vi "Main_Robot.vi"(0 "VISA resource name":refnum<visa-resource-name>="COM1", 1 "baud rate":u32=9600, 4 "data bits":u16=8 min=5 max=8 step=1, 5 "parity":u16(ring) items=["None", "Odd", "Even", "Mark", "Space"], 7 "stop bits":u16(ring)=10 items=["1.0"=10, "1.5"=15, "2.0"=20], 9 "XON Character":u8=17 format="%.0x", 14 "XOFF Character":u8=19 format="%.0x", 15 "timeout (ms)":u32=10000, 21 "End read on termination character?":bool=TRUE, 24 "termination char\n(0xA = '\\n' = LF)":u8=10 format="%.0x", 25 "Input\nbuffer size":u32=4096) -> ()   [LabVIEW 2009]
doc: "The Advanced Serial Read and Write example performs a Serial Port Read, a Serial Port Write, or a combination of these actions while setting some advanced serial features like buffer size, termination characters, and XON/XOFF flow control. The user selects the actions (read or write) on the front panel. If both are selected, the VI will write the data first, read the data and then close the VISA session that is opened to the port. \n\nThe parameters set for the serial port must match the parameters of the connected instrument or device. In this example, the bytes to read parameter specifies the number of bytes that the serial port reads. If there were more bytes at the port than the number specified in bytes to read, those bytes would not be read. Also, if you specify to read more bytes than the number of bytes actually read, you might receive a timeout error message.\n\nINSTRUCTIONS:\n1) Select the serial resource and configuration parameters (baud rate, data bits, parity, stop bits, flow control).\n2) Termination character can be enabled and set. Also, set the required input buffer size prior to running the example.\n3) Select the operations to be performed. \n4) Connect the serial port to your device. If no device is available, perform a loopback test by doing one of the following. Short pins 2 and 3 on a RS-232 cable or short pin 4 to pin 8 and pin 5 to pin 9 on a RS-485/422 cable. \n5) Run the VI to see the data read. (The \"read string\" will match the \"string to write\" if a loopback test was performed.)\n\nThis example exposes several advanced features that you may need for your application. Not all applications need all the features shown in this example. The input buffer size is likely an important setting that you want to control in your application. This example expands upon the flow control option for XON and XOFF, allowing the user to choose those control characters. The timeout parameter has been brought to the front panel so a user can specify the time period the VISA Read will wait for the number of bytes to read before timing out. Also, the user has several controls for the termination character, which is discussed later.\n\nNote that you can press the write and read buttons and change the bytes to read parameters on the fly, while the example is running. However, you must stop the example to change the other configuration parameters after the example has started running, and then run again.\n\nSet the I/O buffer size slightly higher the amount of data you expect to receive. This is very important for applications that don't use flow control, as you may lose characters if the receive buffer overflows.\n\nSetting the timeout period ensures that the operation returns with a timeout error if the operation cannot be performed in the specified time period. \n\nSome devices require a termination character in order to identify the end of command strings. Some devices send a termination character to signify the end of data to be read. \n\nThis example shows how you can end the Read operation once a termination character is detected in the buffer and/or append a termination character at the end of the Write data. To enable the Read to end on a termination character, use the VISA Configure Serial Port or use the VISA Properties Serial End Mode for Reads, Termination Character Enable, and Termination Character. To end the Write with a termination character, use the VISA Properties Serial End Mode for Writes, the Send End Enable, and Termination Character. In this example, the same termination character is used for both the Read and the Write. You can specify two different characters for your application, if desired.\n\nYour application may require specific characters for the XON/XOFF Flow Control. You can specify these characters with the VISA Properties Flow Control XOFF Character and Flow Control XON Character. Note that if the standard XON and XOFF characters are used, then decimal 17 and 19 are unavailable for data values. Remember that using flow control and setting an adequate buffer size allow you to prevent buffer overflows."
uses:
  <vilib>/Instr/_visa.llb/VISA Configure Serial Port (Instr).vi
  <vilib>/measure/madcrms.llb/Basic Averaged DC-RMS for 1 Chan.vi
  <vilib>/express/express analysis/Spectral/XNode/ExpressSpectralMeasurementsBlockNode.xnode
  <vilib>/express/express analysis/Spectral/Block/exnSpectralBlock spectral measurements peak poly.vi
  <vilib>/express/express analysis/Spectral/Block/exnSpectralBlock spectral measurements peak DDT.vi
  <vilib>/measure/NI_MAPro.lvlib
panel:
  in  "Transmit \nInterval (s)":dbl=1.0
  out "Data \nTransmit":string
  in  "I DC":dbl=1.0
  in  "Q DC":dbl=1.0
  out "Human \nDetected?":bool
  in  "Threshold":dbl=200.0
  out "Intensity":waveform(dbl)(graph)
  out "I/Q Spectrum":dynamicdata(graph)
  out "Q channel":waveform(dbl)(graph)={"t0"=timestamp(3198752920.9360003 s since 1904-01-01), "dt"=0.08500000089406967, "Y"=[0.0, 0.0, 0.0, 0.0, 0.0, 0.0, 0.0, 0.0, 0.0, 0.0, 0.0, 0.0, 0.0, 0.0, 0.0, 0.0, 0.0, 0.0, 0.0, 0.0, 0.0, 0.0, 0.0, 0.0, 0.0, 0.0, 0.0, 0.0, 0.0, 0.0, 0.0, 0.0, 0.0, 0.0, 0.0, 0.0, 0.0, 0.0, 0.0, 0.0, 0.0, 0.0, 0.0, 0.0, 0.0, 0.0, 0.0, 0.0, 0.0, 0.0, 0.0, 0.0, 0.0, 0.0, 0.0, 0.0, 0.0, 0.0, 0.0, 0.0, 0.0, 0.0913849025964737, 0.286313533782959, 0.027054062113165855, 0.019259560853242874, 0.2238655835390091, -0.08488079905509949, -0.24375496804714203, -0.09403041750192642, -0.1046101301908493, -0.17000871896743774, 0.13043256103992462, -0.18301288783550262, -0.2802070379257202, -0.05985879898071289, 0.032467812299728394, -0.06909587979316711, 0.12423869222402573, -0.13009318709373474, -0.09696193039417267, 0.13724742829799652, -0.2714601755142212, -0.3184712529182434, 0.13420049846172333, 0.05935952439904213, -0.05841037631034851, 0.2082899808883667, -0.03580809012055397, -0.22062736749649048, 0.06683129817247391, -0.15559138357639313, -0.2515611946582794, 0.05501296743750572, 0.19322194159030914, 0.14264245331287384, 0.36089611053466797, -0.06836720556020737, -0.0454566664993763, -0.0610920712351799, -0.2674013674259186, -0.22359579801559448, -0.09999596327543259, 0.049278225749731064, -0.0071744536980986595, -0.060943424701690674, 0.19243650138378143, 0.10976719856262207, 0.10197310894727707, 0.07962939888238907, 0.2600933611392975, 0.7772611379623413, 0.5951973795890808, 0.4565841257572174, 0.5391018390655518, 0.2501334249973297, -0.05727807804942131, -0.42460599541664124, -0.49300429224967957, -0.6962898373603821, -0.6063411831855774, -0.371660977602005, -0.45583224296569824, -0.3658473789691925, 0.27788665890693665, 0.13202670216560364, -0.05904369801282883, 0.19415463507175446, -0.07230788469314575]}
  out "I channel":waveform(dbl)(graph)={"t0"=timestamp(3198752920.9360003 s since 1904-01-01), "dt"=0.08500000089406967, "Y"=[0.0, 0.0, 0.0, 0.0, 0.0, 0.0, 0.0, 0.0, 0.0, 0.0, 0.0, 0.0, 0.0, 0.0, 0.0, 0.0, 0.0, 0.0, 0.0, 0.0, 0.0, 0.0, 0.0, 0.0, 0.0, 0.0, 0.0, 0.0, 0.0, 0.0, 0.0, 0.0, 0.0, 0.0, 0.0, 0.0, 0.0, 0.0, 0.0, 0.0, 0.0, 0.0, 0.0, 0.0, 0.0, 0.0, 0.0, 0.0, 0.0, 0.0, 0.0, 0.0, 0.0, 0.0, 0.0, 0.0, 0.0, 0.0, 0.0, 0.0, 0.0, 0.0913849025964737, 0.286313533782959, 0.027054062113165855, 0.019259560853242874, 0.2238655835390091, -0.08488079905509949, -0.24375496804714203, -0.09403041750192642, -0.1046101301908493, -0.17000871896743774, 0.13043256103992462, -0.18301288783550262, -0.2802070379257202, -0.05985879898071289, 0.032467812299728394, -0.06909587979316711, 0.12423869222402573, -0.13009318709373474, -0.09696193039417267, 0.13724742829799652, -0.2714601755142212, -0.3184712529182434, 0.13420049846172333, 0.05935952439904213, -0.05841037631034851, 0.2082899808883667, -0.03580809012055397, -0.22062736749649048, 0.06683129817247391, -0.15559138357639313, -0.2515611946582794, 0.05501296743750572, 0.19322194159030914, 0.14264245331287384, 0.36089611053466797, -0.06836720556020737, -0.0454566664993763, -0.0610920712351799, -0.2674013674259186, -0.22359579801559448, -0.09999596327543259, 0.049278225749731064, -0.0071744536980986595, -0.060943424701690674, 0.19243650138378143, 0.10976719856262207, 0.10197310894727707, 0.07962939888238907, 0.2600933611392975, 0.7772611379623413, 0.5951973795890808, 0.4565841257572174, 0.5391018390655518, 0.2501334249973297, -0.05727807804942131, -0.42460599541664124, -0.49300429224967957, -0.6962898373603821, -0.6063411831855774, -0.371660977602005, -0.45583224296569824, -0.3658473789691925, 0.27788665890693665, 0.13202670216560364, -0.05904369801282883, 0.19415463507175446, -0.07230788469314575]}
  out "Hiher2":u8
  out "Lower6":u8
  in  "t0":timestamp=timestamp(3198752888.296 s since 1904-01-01)
  in  "FFT":i32=256
  in  "stop":bool
  in  "flow control":u16(ring) items=["None"=0, "XON/XOFF"=1, "RTS/CTS"=2, "DTR/DSR"=4]
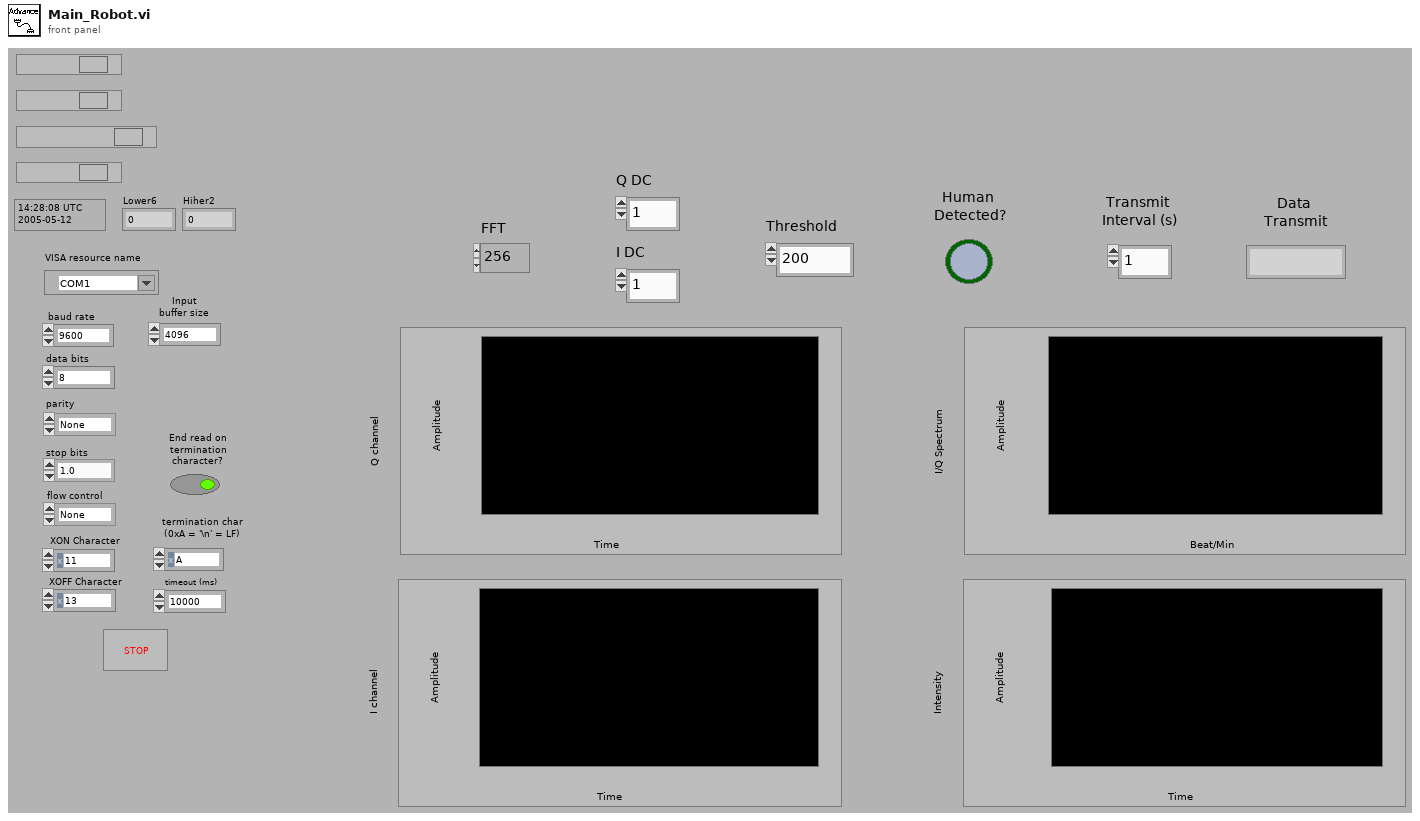
[diagram p1: front panel]
types:
  T1 = cluster{"averaging mode":u16, "weighting mode":u16, "number of averages":u32}
  T2 = cluster{"dB On (F)":bool, "unwrap phase (F)":bool, "convert to degree (F)":bool}
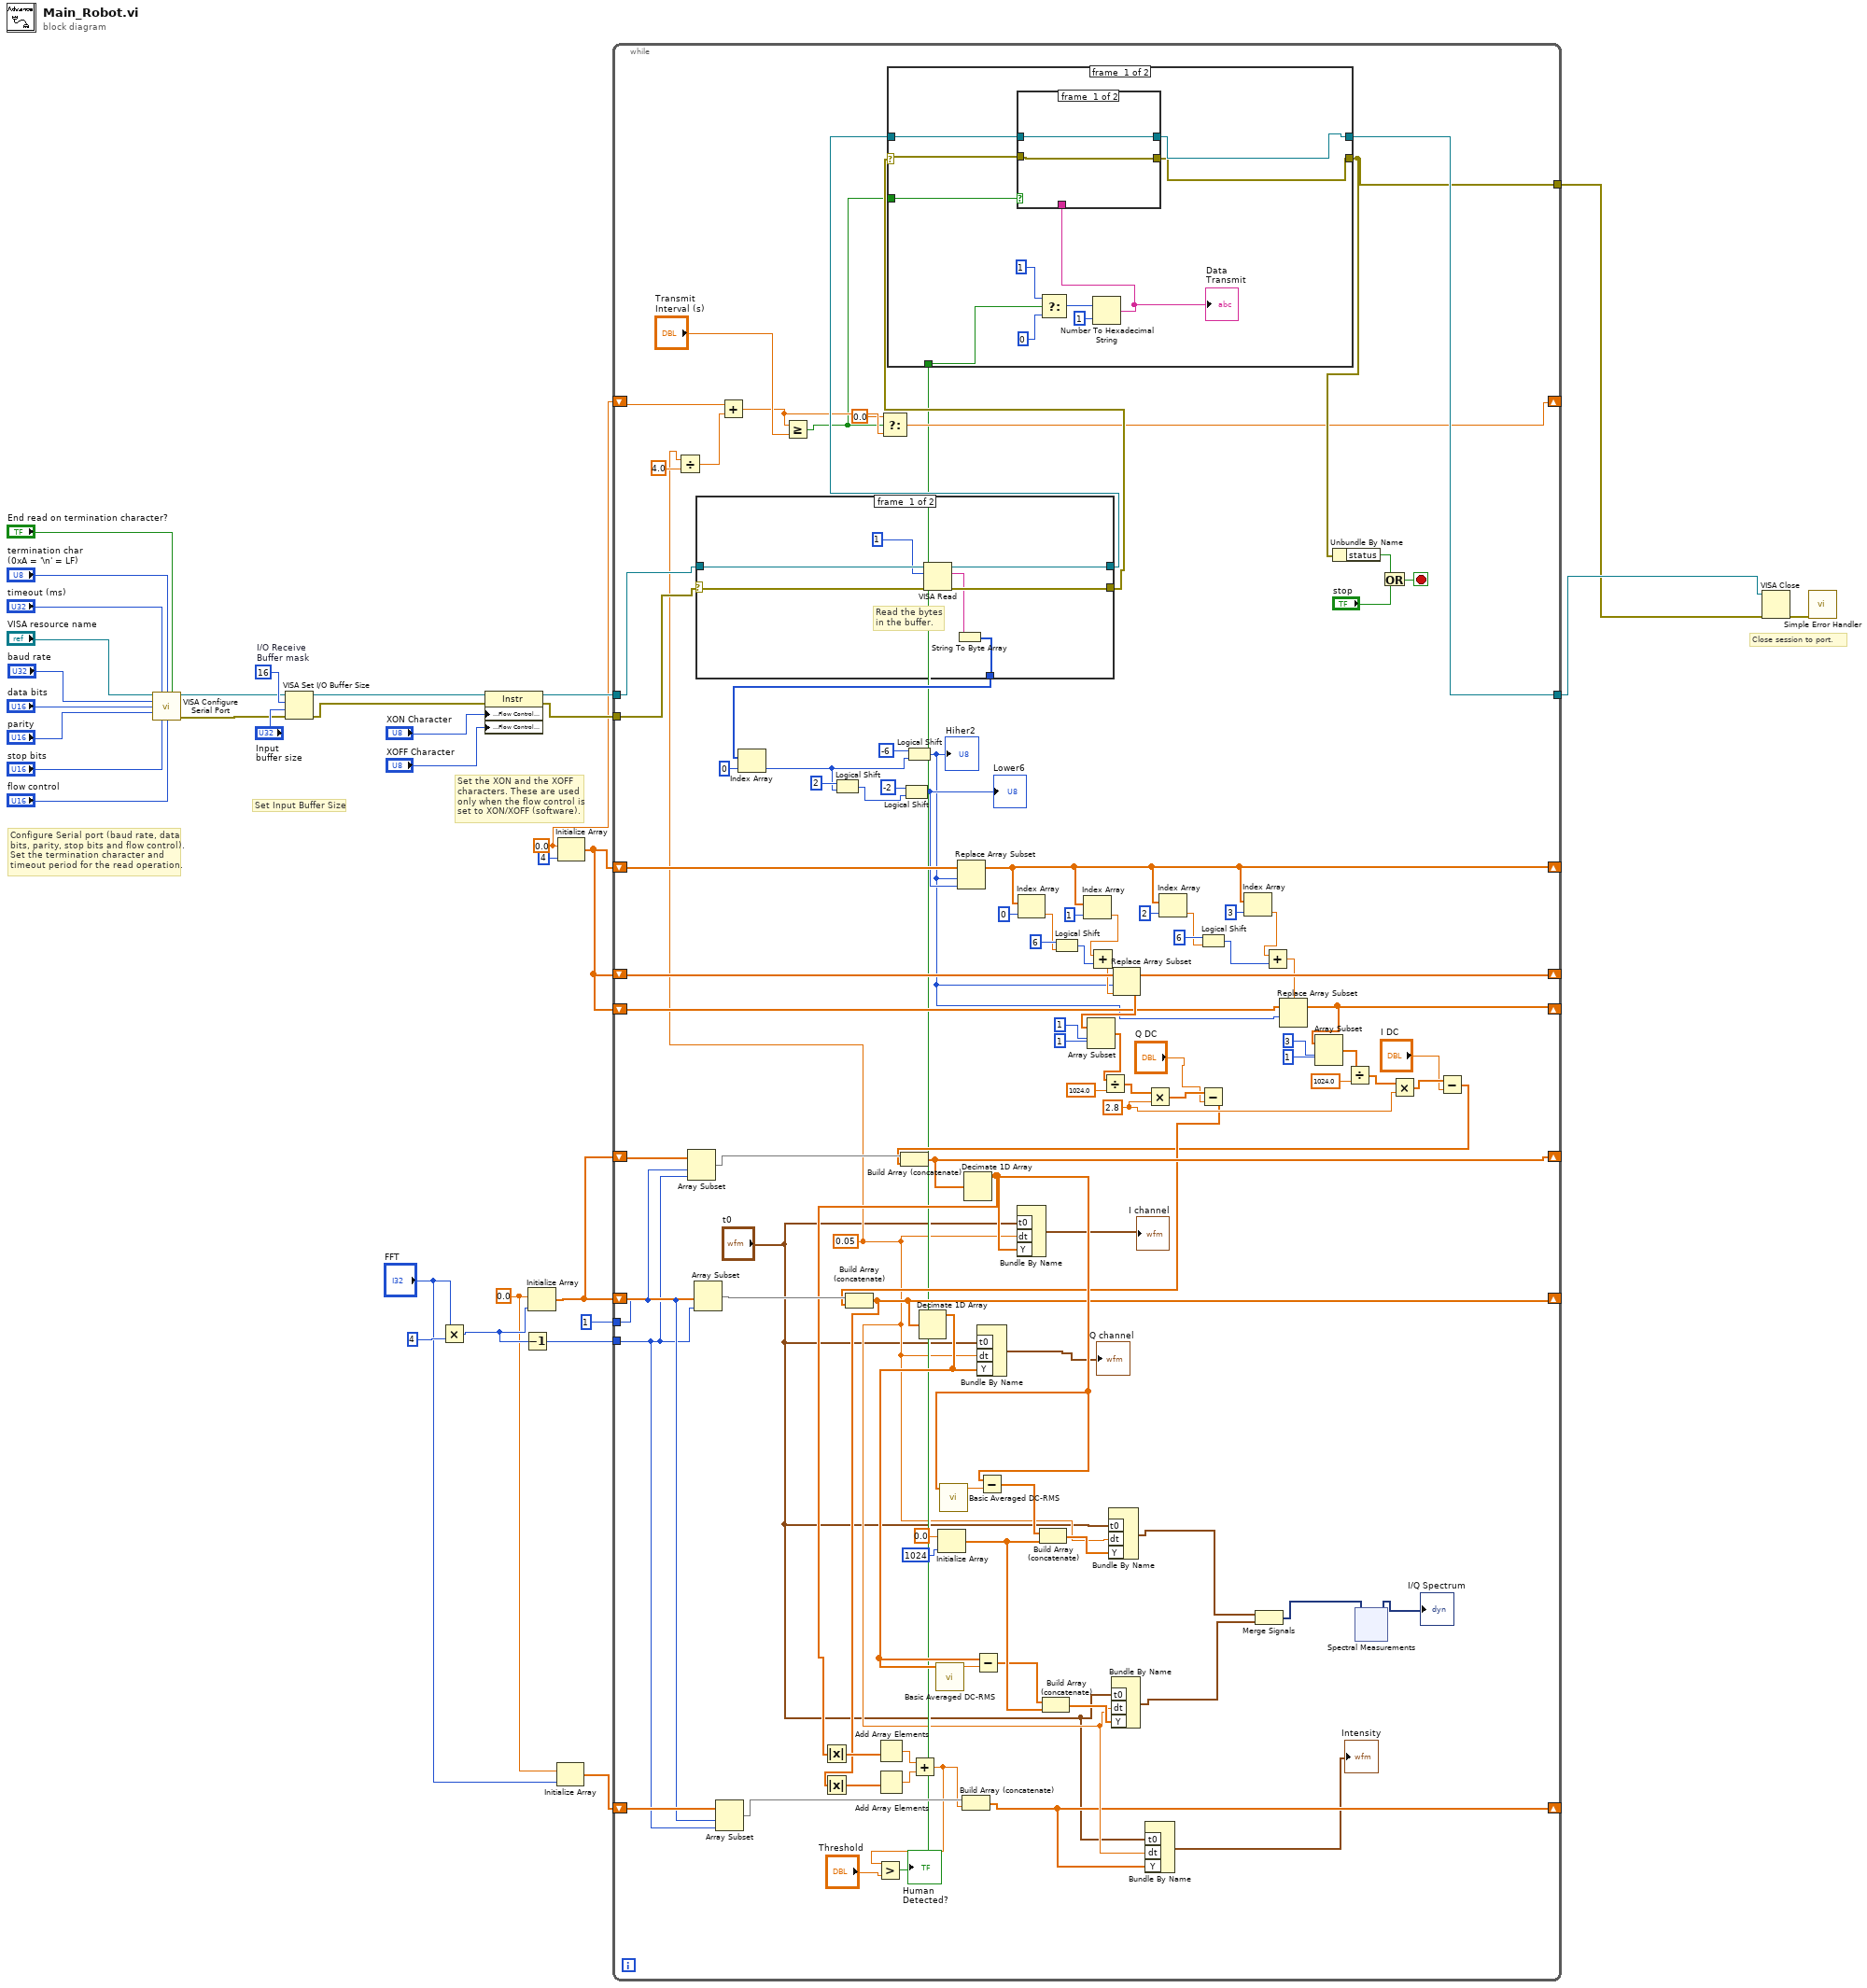
[diagram p0: block diagram]
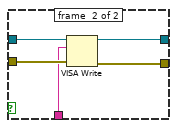
[diagram p2: hidden frame]
diagram:
  w1 = 0.0 ("element")
  w5 = 0.0 ("element")
  w26 = u16 16  # I/O Receive Buffer mask
  # "Set the XON and the XOFF\ncharacters. These are used\nonly when the flow control is\nset to XON/XOFF (software)."
  # "Configure Serial port (baud rate, data\nbits, parity, stop bits and flow control).\nSet the termination character and\ntimeout period for the read operation."
  # "Set Input Buffer Size"
  # "Close session to port."
  n1 = call-poly "VISA Configure Serial Port"("VISA resource name"="VISA resource name", "timeout (10sec)"="timeout (ms)", "termination char\n(0xA = '\\n' = LF)"="termination char\n(0xA = '\\n' = LF)", "Enable Termination\nChar (T)"="End read on termination character?", "baud rate (9600)"="baud rate", "data bits (8)"="data bits", "parity (0:none)"="parity", "stop bits (10: 1 bit)"="stop bits", "flow control (0:none)"="flow control") -> ("VISA resource name out"=w15:refnum<visa-resource-name>, "error out"=w14:errorcluster)  [unwired: 5 in]
  n2 = VISA Set I/O Buffer Size(VISA resource name=w15, mask (16)=w26, size (4096)="Input\nbuffer size", error in (no error)=w14) -> (VISA resource name out=w22:refnum<visa-resource-name>, error out=w21:errorcluster)
  n3 = Multiply(x="FFT", y=4) -> (x*y=w8:i32)
  n4 = property class="Instr"(reference=w22, error in=w21, "Serial Settings:Flow Control XON Character"="XON Character", "Serial Settings:Flow Control XOFF Character"="XOFF Character") -> (reference out=w16:refnum<visa-resource-name>, error out=w18:errorcluster)
  n5 = Decrement(x=w8) -> (x-1=w13:i32)
  n6 = Initialize Array(w5, w8) -> (w10:dbl[])
  n7 = Initialize Array(w5, "FFT") -> (w4:dbl[])
  n8 = Initialize Array(w1, 4 ("dimension size")) -> (w9:dbl[])
  n9 = while {
    tunnel: w18 -> [w53]
    tunnel: w16 -> [w54]
    tunnel: [w50] -> w3
    tunnel: w13 -> [w35]
    tunnel: 1 ("index") -> [w36]
    shift-right: [w66] -> _
    shift-left: w10 -> [w129]
    shift-right: [w117] -> _
    shift-left: w9 -> [w123]
    shift-right: [w70] -> _
    shift-left: w10 -> [w107]
    shift-right: [w99] -> _
    shift-left: w9 -> [w101]
    shift-right: [w91] -> _
    shift-left: w9 -> [w94]
    shift-right: [w39] -> _
    shift-left: w4 -> [w73]
    tunnel: [w49] -> w2
    shift-right: [w44] -> _
    shift-left: w1 -> [w48]
    stop <- w133 stop-if-true
    w78 = 2.8 ("y")
    w40 = 0.05 ("dt")
    n10 = Divide(x=w40, y=4.0) -> (x/y=w42:dbl)
    n11 = Array Subset(array=w107, index=w36, length=w35) -> (w108:dbl[])
    n12 = Array Subset(array=w129, index=w36, length=w35) -> (w131:dbl[])
    n13 = case "Read bytes from port." shown="No Error" w53 {
      selector: w53 -> [w169 w174]
      tunnel: [w171 w174] -> w51
      tunnel: [w172 w175] -> w52
      tunnel: w54 -> [w170 w175]
      tunnel: [w167 u8[] [] ("unsigned byte array")] -> w106
      frame #0 {
        # "Read the bytes\nin the buffer."
        n14 = VISA Read(VISA resource name=w170, byte count=u32 1, error in (no error)=w169) -> (VISA resource name out=w172:refnum<visa-resource-name>, read buffer=w168:string, error out=w171:errorcluster)  [unwired: 1 out]
        n15 = String To Byte Array(string=w168) -> (unsigned byte array=w167:u8[])
      }
      frame #1 {
        # "Error occurred \nreading Bytes at \nSerial Port"
      }
    }
    n16 = Array Subset(array=w73, index=w36, length=w35) -> (w72:dbl[])
    n17 = Add(x=w48, y=w42) -> (x+y=w46:dbl)
    n18 = Index Array(array=w106, index=0) -> (element=w126:u8)
    n19 = Greater Or Equal?(x=w46, y="Transmit \nInterval (s)") -> (x >= y?=w34:bool)
    n20 = Logical Shift(y=i8 2, x=w126) -> (x << y=w125:u8)
    n21 = Select(t=0.0, s=w34, f=w46) -> (s? t:f=w44:dbl)
    n22 = Logical Shift(y=i8 -2, x=w125) -> (x << y=w122:u8)
    "Lower6" <- w122
    n23 = Logical Shift(y=i8 -6, x=w126) -> (x << y=w89:u8)
    "Hiher2" <- w89
    n24 = Initialize Array(0.0 ("element"), 1024 ("dimension size")) -> (w82:dbl[])
    n25 = Replace Array Subset(array=w123, new element=w122, index=w89) -> (w117:dbl[])
    n26 = Index Array(array=w117, index=0) -> (element=w115:dbl)
    n27 = Logical Shift(y=i16 6, x=w115) -> (x << y=w111:u32)
    n28 = Index Array(array=w117, index=1) -> (element=w112:dbl)
    n29 = Add(x=w112, y=w111) -> (x+y=w100:dbl)
    n30 = Replace Array Subset(array=w101, new element=w100, index=w89) -> (w99:dbl[])
    n31 = Array Subset(array=w99, index=1, length=1) -> (w96:dbl[])
    n32 = Divide(x=w96, y=1024.0) -> (x/y=w104:dbl[])
    n33 = Multiply(x=w104, y=w78) -> (x*y=w60:dbl[])
    n34 = Index Array(array=w117, index=2) -> (element=w113:dbl)
    n35 = Logical Shift(y=i16 6, x=w113) -> (x << y=w109:u32)
    n36 = Subtract(x=w60, y="Q DC") -> (x-y=w59:dbl[])
    n37 = Build Array (concatenate)(w131, w59) -> (w66:dbl[])
    n38 = Absolute Value(x=w66) -> (abs(x)=w76:dbl[])
    n39 = Add Array Elements(numeric array=w76) -> (sum=w74:dbl)
    n40 = Decimate 1D Array(w66) -> (w65:dbl[])  [unwired: 3 out]
    n41 = call-poly <vilib>:"Basic Averaged DC-RMS.vi"("signal in"=w65) -> ("DC value"=w81:dbl)  [unwired: 7 in, 3 out]
    n42 = Subtract(x=w65, y=w81) -> (x-y=w80:dbl[])
    n43 = Bundle By Name("t0"="t0", "dt"=w40, "Y"=w65) -> (→"Q channel":waveform(dbl))  [unwired: 1 in]
    n44 = Build Array (concatenate)(w80, w82) -> (w83:dbl[])
    n45 = Bundle By Name("t0"="t0", "dt"=w40, "Y"=w83) -> (w64:waveform(dbl))  [unwired: 1 in]
    n46 = Index Array(array=w117, index=3) -> (element=w110:dbl)
    n47 = Add(x=w110, y=w109) -> (x+y=w95:dbl)
    n48 = Replace Array Subset(array=w94, new element=w95, index=w89) -> (w91:dbl[])
    n49 = Array Subset(array=w91, index=3, length=1) -> (w90:dbl[])
    n50 = Divide(x=w90, y=1024.0) -> (x/y=w102:dbl[])
    n51 = Multiply(x=w102, y=w78) -> (x*y=w58:dbl[])
    n52 = Subtract(x=w58, y="I DC") -> (x-y=w57:dbl[])
    n53 = Build Array (concatenate)(w108, w57) -> (w70:dbl[])
    n54 = Decimate 1D Array(w70) -> (w71:dbl[])  [unwired: 3 out]
    n55 = Absolute Value(x=w71) -> (abs(x)=w77:dbl[])
    n56 = Add Array Elements(numeric array=w77) -> (sum=w75:dbl)
    n57 = Add(x=w75, y=w74) -> (x+y=w62:dbl)
    n58 = Greater?(x=w62, y="Threshold") -> (0:w41:bool)
    "Human \nDetected?" <- w41
    n59 = case "Read bytes from port." shown="No Error" w51 {
      selector: w51 -> [w155 w164]
      tunnel: [w148 w164] -> w49
      tunnel: [w149 w165] -> w50
      tunnel: w52 -> [w156 w165]
      tunnel: w41 -> [w147 _]
      tunnel: w34 -> [w146 _]
      frame #0 {
        n60 = Select(t=1, s=w147, f=u8 0) -> (s? t:f=w152:i32)
        n61 = Number To Hexadecimal String(1:i16 1 ("width (-)"), 2:w152) -> (0:w150:string)
        "Data \nTransmit" <- w150
        n62 = case shown="True" w146 {
          tunnel: w156 -> [w158 w163]
          tunnel: w155 -> [w157 w162]
          tunnel: [w158 w161] -> w149
          tunnel: [w157 w160] -> w148
          tunnel: w150 -> [_ w159]
          frame #0 {
          }
          frame #1 {
            n63 = VISA Write(VISA resource name=w163, write buffer=w159, error in (no error)=w162) -> (VISA resource name out=w161:refnum<visa-resource-name>, error out=w160:errorcluster)  [unwired: 1 out]
          }
        }
      }
      frame #1 {
        # "Error occurred \nreading Bytes at \nSerial Port"
      }
    }
    n64 = call-poly <vilib>:"Basic Averaged DC-RMS.vi"("signal in"=w71) -> ("DC value"=w85:dbl)  [unwired: 7 in, 3 out]
    n65 = Build Array (concatenate)(w72, w62) -> (w39:dbl[])
    n66 = Subtract(x=w71, y=w85) -> (x-y=w84:dbl[])
    n67 = Bundle By Name("t0"="t0", "dt"=w40, "Y"=w71) -> (→"I channel":waveform(dbl))  [unwired: 1 in]
    n68 = Build Array (concatenate)(w84, w82) -> (w68:dbl[])
    n69 = Bundle By Name("t0"="t0", "dt"=w40, "Y"=w68) -> (w67:waveform(dbl))  [unwired: 1 in]
    n70 = Bundle By Name("t0"="t0", "dt"=w40, "Y"=w39) -> (→"Intensity":waveform(dbl))  [unwired: 1 in]
    n71 = Merge Signals(w67, w64) -> (w79:dynamicdata)
    n72 = Unbundle By Name(w49) -> ("status"=w134:bool)
    n73 = xnode "Spectral Measurements"("Signals"=w79) -> ("FFT - (Peak)"=→"I/Q Spectrum":dynamicdata)  [unwired: 2 in, 3 out]
    n74 = Or(x=w134, y="stop") -> (x .or. y?=w133:bool)
  }
  n75 = VISA Close(VISA resource name=w3, error in (no error)=w2) -> (error out=w31:errorcluster)
  n76 = call <vilib>:"Simple Error Handler.vi"("error in (no error)"=w31) -> ()  [unwired: 4 in, 5 out]
